vi "templates COLUMNS data keys.vi"(9 "Template Keys":T1, 10 "HTM Keys":T1) -> (2 "HTM Keys":T1)   [LabVIEW 2011]
uses:
  ITK EXT/utils/keyedarr.llb/Keyed Array.ctl
  ITK EXT/utils/strutil.llb/Case Matching.ctl
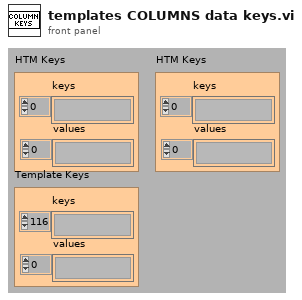
[diagram p1: front panel]
types:
  T1 = typedef "Keyed Array.ctl" = cluster{"keys":string[], "values":string[]}
  T2 = typedef "Case Matching.ctl" = enum16{"a != A", "a == A", "system"}
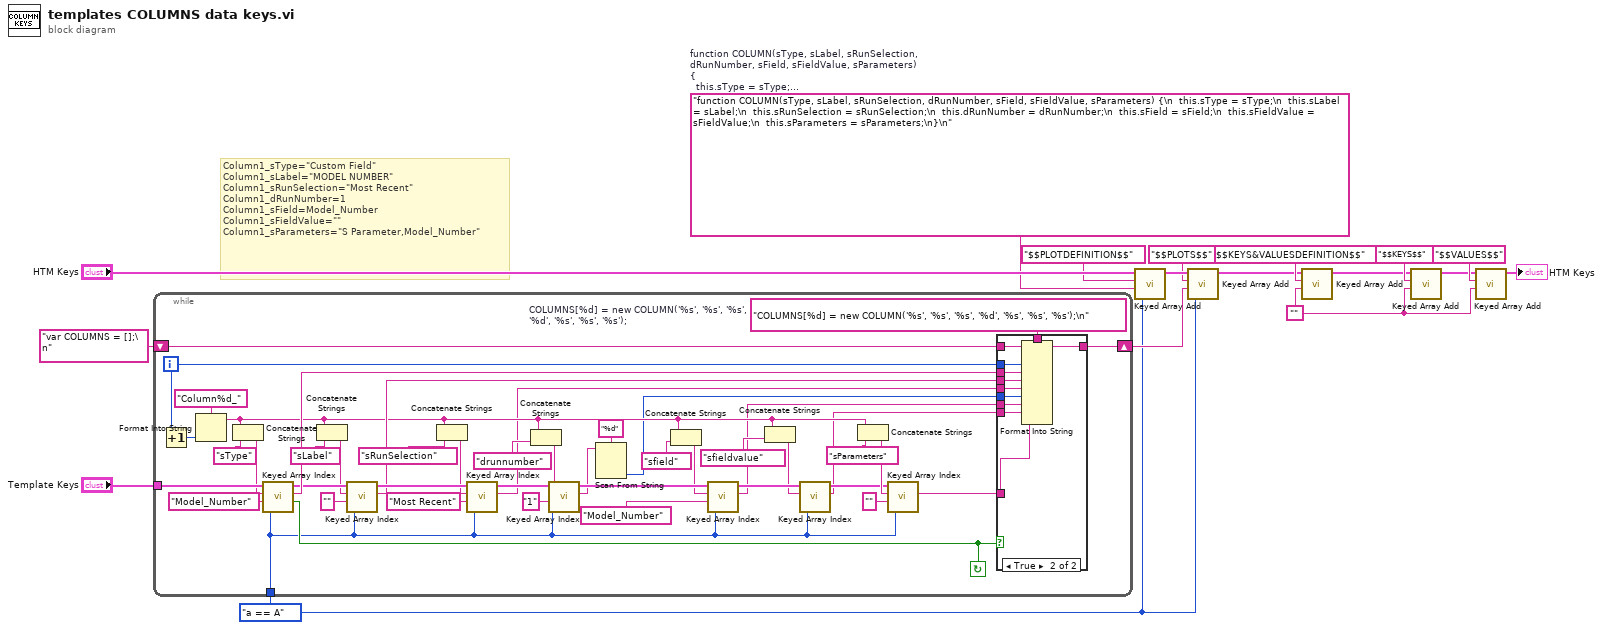
[diagram p0: block diagram]
diagram:
  w1 = ""
  w9 = Case_Matching."a == A" ("case matching (sensitive)")
  w14 = "function COLUMN(sType, sLabel, sRunSelection, dRunNumber, sField, sFieldValue, sParameters) {\n  this.sType = sType;\n  this.sLabel = sLabel;\n  this.sRunSelection = sRunSelection;\n  this.dRunNumber = dRunNumber;\n  this.sField = sField;\n  this.sFieldValue = sFieldValue;\n  this.sParameters = sParameters;\n}\n"  # function COLUMN(sType, sLabel, sRunSelection, dRunNumber, sField, sFieldValue, sParameters) {   this.sType = sType;   this.sLabel = sLabel;   this.sRunSelection = sRunSelection;   this.dRunNumber = dRunNumber;   this.sField = sField;   this.sFieldValue = sFieldValue;   this.sParameters = sParameters; }
  # "Column1_sType=\"Custom Field\"\nColumn1_sLabel=\"MODEL NUMBER\"\nColumn1_sRunSelection=\"Most Recent\"\nColumn1_dRunNumber=1\nColumn1_sField=Model_Number\nColumn1_sFieldValue=\"\"\nColumn1_sParameters=\"S Parameter,Model_Number\""
  n1 = while {
    shift-right: [w60] -> w11
    shift-left: "var COLUMNS = [];\n" ("format string") -> [w61]
    tunnel: "Template Keys" -> [w47]
    tunnel: w9 -> [w30]
    i -> [w41]
    stop <- w38 continue-if-true
    w62 = "COLUMNS[%d] = new COLUMN('%s', '%s', '%s', '%d', '%s', '%s', '%s');\n"  # COLUMNS[%d] = new COLUMN('%s', '%s', '%s', '%d', '%s', '%s', '%s');
    n2 = Increment(x=w41) -> (x+1=w40:i32)
    n3 = Format Into String(format string="Column%d_", w40) -> (resulting string=w37:string)  [unwired: 2 in, 1 out]
    n4 = Concatenate Strings(w37, "sType" ("format string")) -> (w46:string)
    n5 = call "Keyed Array Index.vi"("case matching (sensitive)"=w30, "default value"="Model_Number", "key"=w46, "array in"=w47) -> ("valid key"=w38:bool, "value"=w56:string, "duplicate array"=w55:T1)  [unwired: 1 out]
    n6 = Concatenate Strings(w37, "sLabel" ("format string")) -> (w45:string)
    n7 = call "Keyed Array Index.vi"("case matching (sensitive)"=w30, "default value"="", "key"=w45, "array in"=w55) -> ("value"=w42:string, "duplicate array"=w51:T1)  [unwired: 2 out]
    n8 = Concatenate Strings(w37, "sRunSelection" ("format string")) -> (w44:string)
    n9 = call "Keyed Array Index.vi"("case matching (sensitive)"=w30, "default value"="Most Recent" ("format string"), "key"=w44, "array in"=w51) -> ("value"=w23:string, "duplicate array"=w32:T1)  [unwired: 2 out]
    n10 = Concatenate Strings(w37, "drunnumber" ("format string")) -> (w31:string)
    n11 = call "Keyed Array Index.vi"("case matching (sensitive)"=w30, "default value"="1", "key"=w31, "array in"=w32) -> ("value"=w21:string, "duplicate array"=w36:T1)  [unwired: 2 out]
    n12 = Scan From String(format string="%d", input string=w21) -> (output 1=w20:i32)  [unwired: 2 in, 4 out]
    n13 = Concatenate Strings(w37, "sfield" ("format string")) -> (w26:string)
    n14 = call "Keyed Array Index.vi"("case matching (sensitive)"=w30, "default value"="Model_Number" ("format string"), "key"=w26, "array in"=w36) -> ("value"=w19:string, "duplicate array"=w35:T1)  [unwired: 2 out]
    n15 = Concatenate Strings(w37, "sfieldvalue" ("format string")) -> (w24:string)
    n16 = call "Keyed Array Index.vi"("case matching (sensitive)"=w30, "key"=w24, "array in"=w35) -> ("value"=w18:string, "duplicate array"=w34:T1)  [unwired: 1 in, 2 out]
    n17 = Concatenate Strings(w37, "sParameters" ("format string")) -> (w43:string)
    n18 = call "Keyed Array Index.vi"("case matching (sensitive)"=w30, "default value"="" ("format string"), "key"=w43, "array in"=w34) -> ("value"=w39:string)  [unwired: 3 out]
    n19 = case shown="True" w38 {
      tunnel: w62 -> [_ w74]
      tunnel: w61 -> [w63 w73]
      tunnel: [w63 w72] -> w60
      tunnel: w56 -> [_ w71]
      tunnel: w42 -> [_ w70]
      tunnel: w41 -> [_ w69]
      tunnel: w20 -> [_ w68]
      tunnel: w19 -> [_ w67]
      tunnel: w18 -> [_ w66]
      tunnel: w39 -> [_ w65]
      tunnel: w23 -> [_ w64]
      frame False {
      }
      frame True {
        n20 = Format Into String(format string=w74, initial string=w73, w69, w71, w70, w64, w68, w67, w66, w65) -> (resulting string=w72:string)  [unwired: 1 in, 1 out]
      }
    }
  }
  n21 = call "Keyed Array Add.vi"("case matching (sensitive)"=w9, "value"=w14, "key"="$$PLOTDEFINITION$$", "array in"="HTM Keys") -> ("array out"=w13:T1)  [unwired: 3 out]
  n22 = call "Keyed Array Add.vi"("case matching (sensitive)"=w9, "value"=w11, "key"="$$PLOTS$$", "array in"=w13) -> ("array out"=w2:T1)  [unwired: 3 out]
  n23 = call "Keyed Array Add.vi"("value"=w1, "key"="$$KEYS&VALUESDEFINITION$$", "array in"=w2) -> ("array out"=w5:T1)  [unwired: 1 in, 3 out]
  n24 = call "Keyed Array Add.vi"("value"=w1, "key"="$$KEYS$$", "array in"=w5) -> ("array out"=w4:T1)  [unwired: 1 in, 3 out]
  n25 = call "Keyed Array Add.vi"("value"=w1, "key"="$$VALUES$$", "array in"=w4) -> ("array out"=→"HTM Keys":T1)  [unwired: 1 in, 3 out]
